vi "intervaloespejo.vi"(6 "tipo":enum16{"manual", "barrido"}(ring), 7 "intervalo":dbl, 8 "fin y":dbl, 9 "fin x":dbl, 10 "inicio y":dbl, 11 "inicio x":dbl) -> (2 "salida":string[](array[string]))   [LabVIEW 2016]
doc: "Este subVI funiciona para crear la cadena de la secuencia de coordenadas a las que se tiene que mover el spot.\n\nA este subVI tiene como entradas la posición actual del spot en x y y, la posición final en x y y, un enom en donde se especifica si se quiere realizar un barrido o medir en una sola posición y el tamaño de paso que se desea realizar.\n\nComo salida tiene un arreglo de tipo string con las posiciones en las que se tiene que mover el spot del láser."
panel:
  out "Array 2":dbl[](array[numeric])
  out "Array":dbl[](array[numeric])
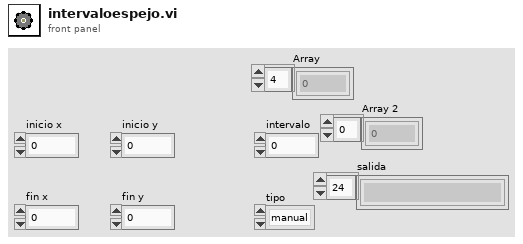
[diagram p1: front panel]
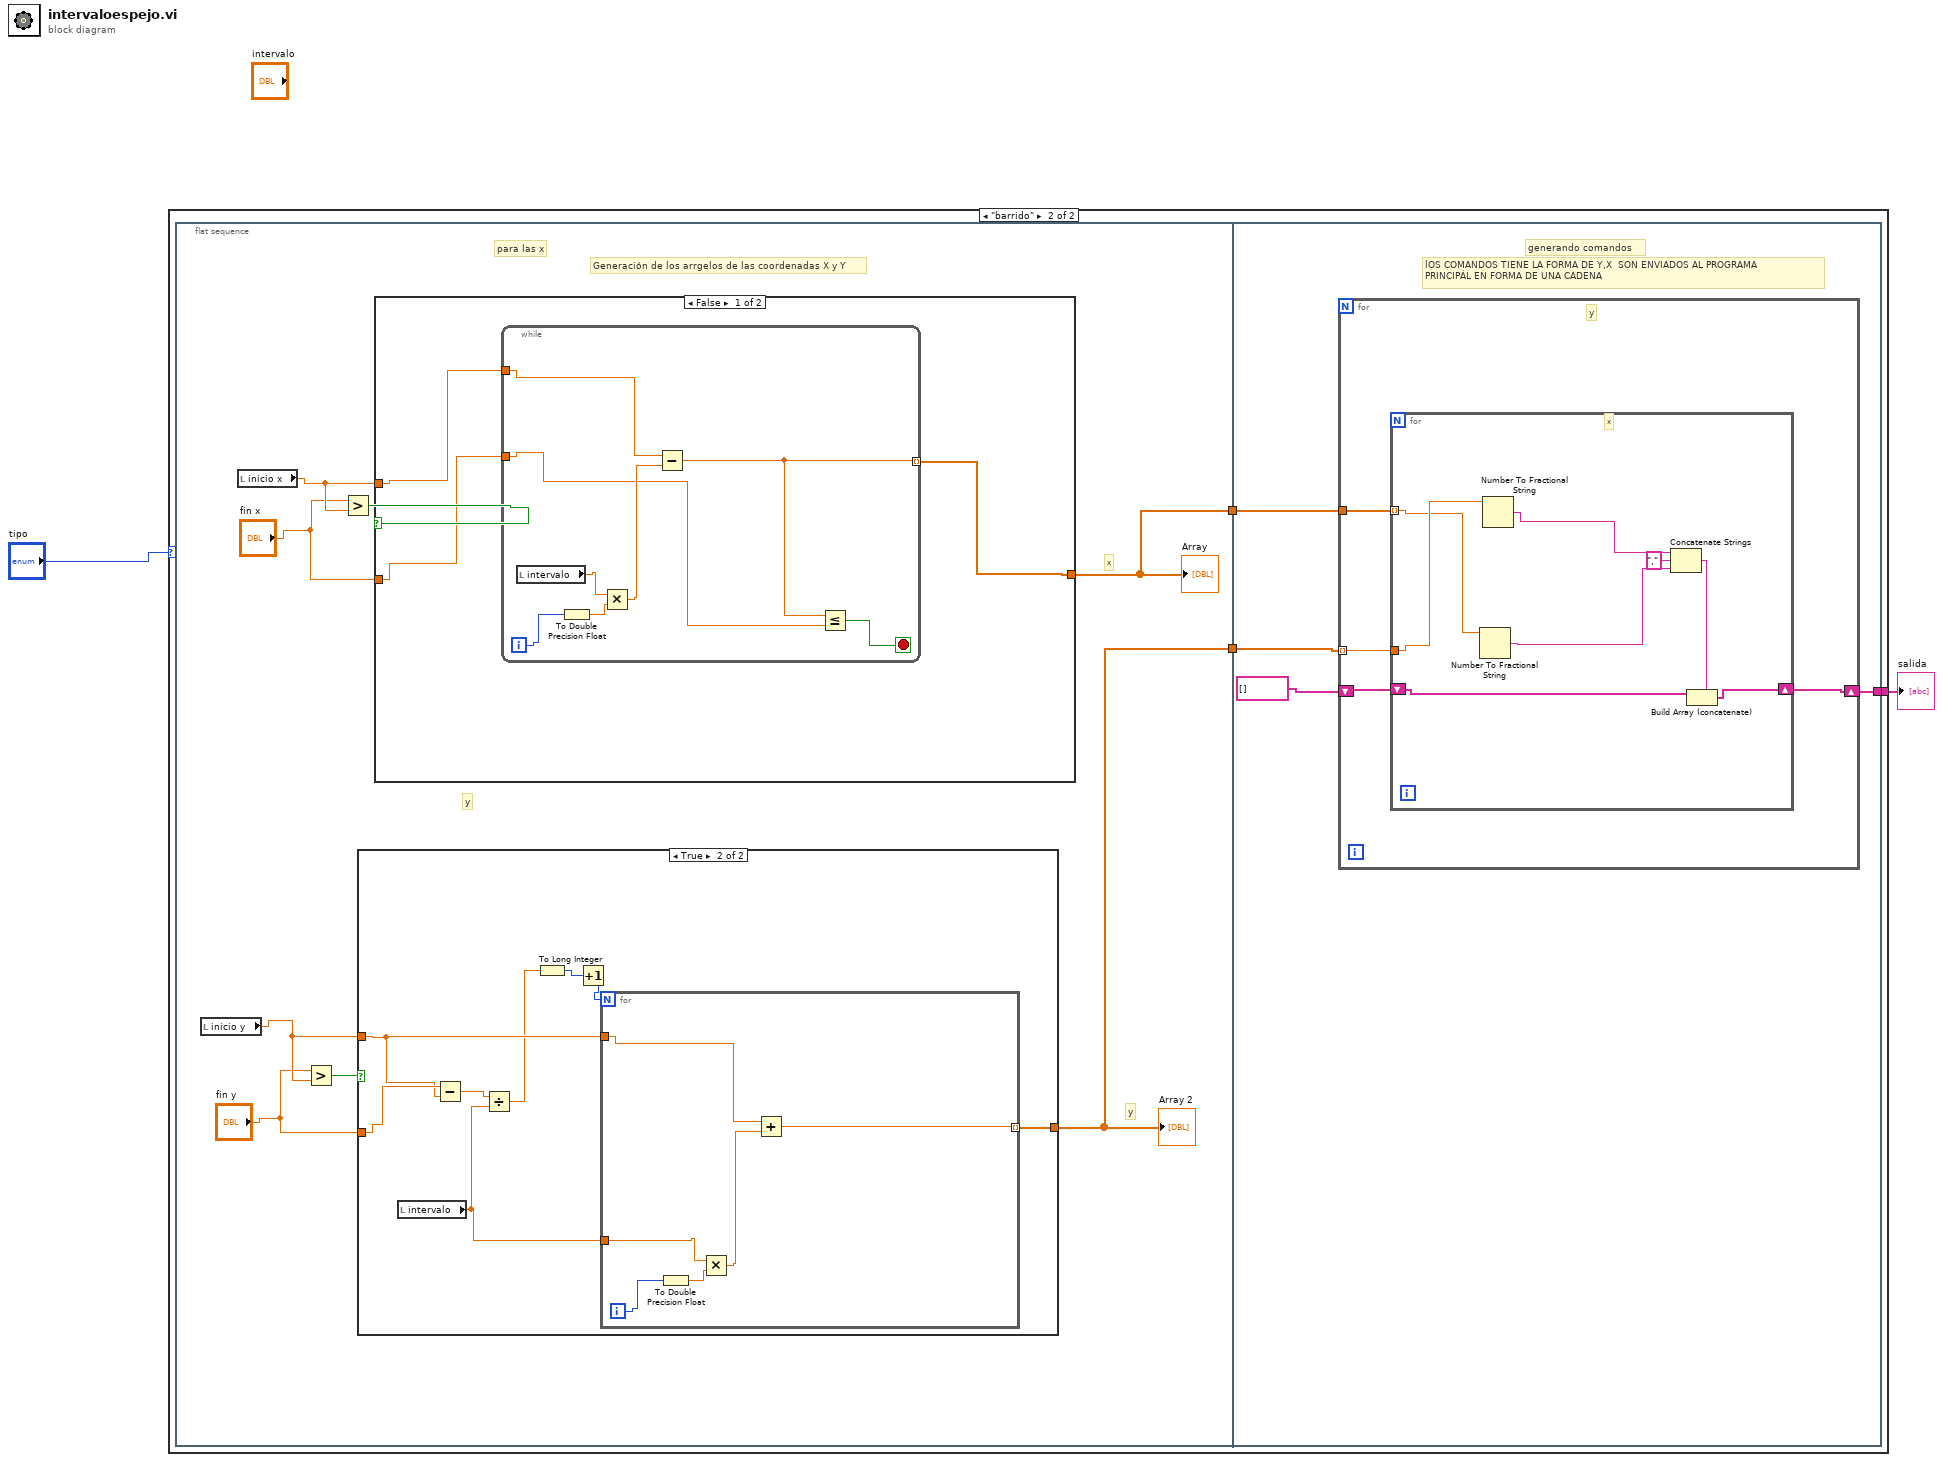
[diagram p0: block diagram]
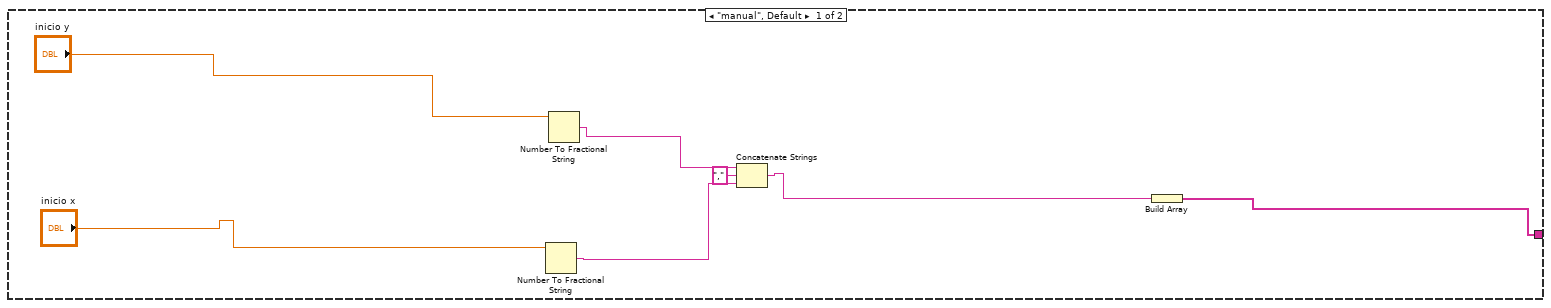
[diagram p2: hidden frame]
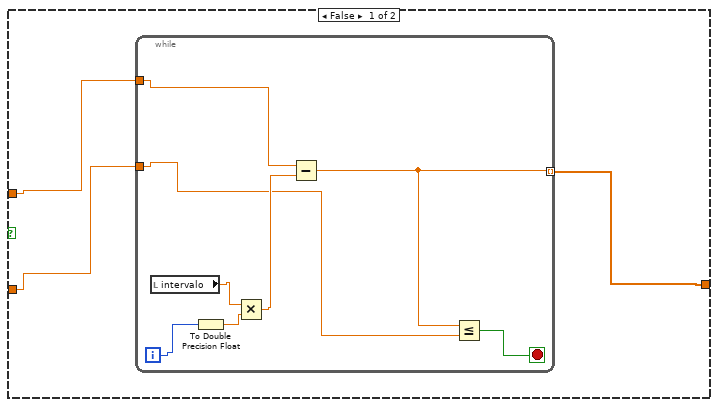
[diagram p3: hidden frame]
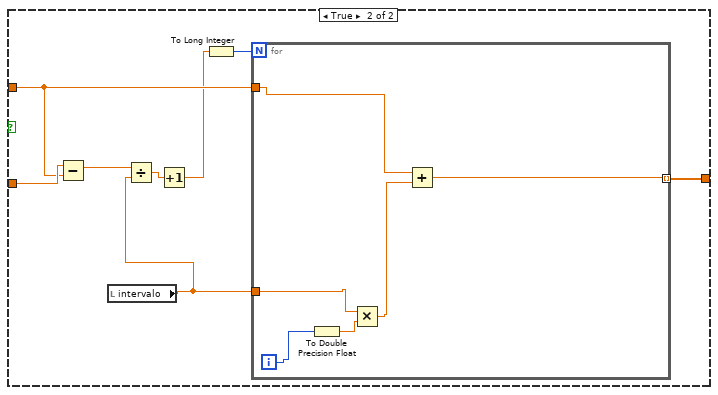
[diagram p4: hidden frame]
diagram:
  n1 = case shown="\"barrido\"" "tipo" {
    tunnel: [w3 w10] -> w1
    frame "manual", Default {
      n2 = Number To Fractional String(number="inicio x") -> (F-format string=w6:string)  [unwired: 3 in]
      n3 = Number To Fractional String(number="inicio y") -> (F-format string=w7:string)  [unwired: 3 in]
      n4 = Concatenate Strings(w7, "," ("string"), w6) -> (w4:string)
      n5 = Build Array(w4) -> (w3:string[])
    }
    frame "barrido" {
      n6 = flat-sequence {
        tunnel: [w14] -> w12
        tunnel: [w13] -> w11
        tunnel: w12 -> [w74]
        tunnel: w11 -> [w73]
        tunnel: [w72] -> w10
        frame #0 {
          # "Generación de los arrgelos de las coordenadas X y Y"
          # "y"
          # "x"
          # "y"
          # "para las x"
          n7 = local read "inicio y"() -> (w16:dbl)
          n8 = local read "inicio x"() -> (w19:dbl)
          n9 = Greater?(x="fin y", y=w16) -> (0:w17:bool)
          n10 = Greater?(x="fin x", y=w19) -> (0:w20:bool)
          n11 = case shown="True" w17 {
            tunnel: w16 -> [w23 w35]
            tunnel: "fin y" -> [w22 w38]
            tunnel: [w21 w39] -> w13
            frame False {
              n12 = while {
                tunnel: w23 -> [w28]
                tunnel: w22 -> [w24]
                tunnel: [w25] -> w21 mode=indexing
                i -> [w29]
                stop <- w26 stop-if-true
                n13 = local read "intervalo"() -> (w31:dbl)
                n14 = To Double Precision Float(number=w29) -> (double precision float=w30:dbl)
                n15 = Multiply(x=w31, y=w30) -> (x*y=w27:dbl)
                n16 = Subtract(x=w28, y=w27) -> (x-y=w25:dbl)
                n17 = Less Or Equal?(x=w25, y=w24) -> (x <= y?=w26:bool)
              }
            }
            frame True {
              n18 = local read "intervalo"() -> (w36:dbl)
              n19 = Subtract(x=w38, y=w35) -> (x-y=w37:dbl)
              n20 = Divide(x=w37, y=w36) -> (x/y=w34:dbl)
              n21 = To Long Integer(number=w34) -> (32bit integer=w33:i32)
              n22 = Increment(x=w33) -> (x+1=w32:i32)
              n23 = for {
                N: w32 -> [_]
                tunnel: w35 -> [w43]
                tunnel: [w41] -> w39 mode=indexing
                tunnel: w36 -> [w40]
                i -> [w44]
                n24 = To Double Precision Float(number=w44) -> (double precision float=w45:dbl)
                n25 = Multiply(x=w40, y=w45) -> (x*y=w42:dbl)
                n26 = Add(x=w43, y=w42) -> (x+y=w41:dbl)
              }
            }
          }
          "Array 2" <- w13
          n27 = case shown="False" w20 {
            tunnel: w19 -> [w48 w62]
            tunnel: "fin x" -> [w47 w63]
            tunnel: [w46 w64] -> w14
            frame False {
              n28 = while {
                tunnel: w48 -> [w53]
                tunnel: w47 -> [w49]
                tunnel: [w50] -> w46 mode=indexing
                i -> [w54]
                stop <- w51 stop-if-true
                n29 = local read "intervalo"() -> (w56:dbl)
                n30 = To Double Precision Float(number=w54) -> (double precision float=w55:dbl)
                n31 = Multiply(x=w56, y=w55) -> (x*y=w52:dbl)
                n32 = Subtract(x=w53, y=w52) -> (x-y=w50:dbl)
                n33 = Less Or Equal?(x=w50, y=w49) -> (x <= y?=w51:bool)
              }
            }
            frame True {
              n34 = Subtract(x=w63, y=w62) -> (x-y=w61:dbl)
              n35 = local read "intervalo"() -> (w60:dbl)
              n36 = Divide(x=w61, y=w60) -> (x/y=w59:dbl)
              n37 = Increment(x=w59) -> (x+1=w57:dbl)
              n38 = To Long Integer(number=w57) -> (32bit integer=w58:i32)
              n39 = for {
                N: w58 -> [_]
                tunnel: w62 -> [w68]
                tunnel: [w66] -> w64 mode=indexing
                tunnel: w60 -> [w65]
                i -> [w69]
                n40 = To Double Precision Float(number=w69) -> (double precision float=w70:dbl)
                n41 = Multiply(x=w65, y=w70) -> (x*y=w67:dbl)
                n42 = Add(x=w68, y=w67) -> (x+y=w66:dbl)
              }
            }
          }
          "Array" <- w14
        }
        frame #1 {
          # "lOS COMANDOS TIENE LA FORMA DE Y,X  SON ENVIADOS AL PROGRAMA \nPRINCIPÁL EN FORMA DE UNA CADENA"
          # "generando comandos"
          n43 = for {
            tunnel: w74 -> [w78]
            tunnel: w73 -> [w77] mode=indexing
            shift-right: [w75] -> w72
            shift-left: string[] [] -> [w76]
            # "y"
            n44 = for {
              tunnel: w78 -> [w82] mode=indexing
              tunnel: w77 -> [w83]
              shift-right: [w80] -> w75
              shift-left: w76 -> [w81]
              # "x"
              n45 = Number To Fractional String(number=w82) -> (F-format string=w85:string)  [unwired: 3 in]
              n46 = Number To Fractional String(number=w83) -> (F-format string=w86:string)  [unwired: 3 in]
              n47 = Concatenate Strings(w86, "," ("string"), w85) -> (w79:string)
              n48 = Build Array (concatenate)(w81, w79) -> (w80:string[])
            }
          }
        }
      }
    }
  }
  "salida" <- w1
